vi "Get_Temperature_Percent.vi"(1 "Temperature":dbl, 2 "Setpoint":dbl) -> (0 "Temperature Percent":dbl)   [LabVIEW 2011]
doc: "This VI is a simple macro that determines an absolute percentage value, correlating to the distance from the current setpoint."
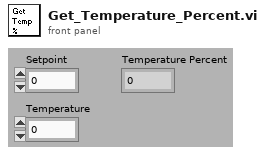
[diagram p1: front panel]
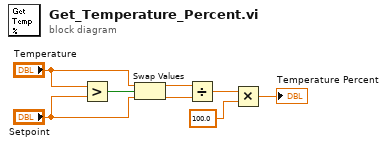
[diagram p0: block diagram]
diagram:
  n1 = Greater?(x="Temperature", y="Setpoint") -> (0:w8:bool)
  n2 = Swap Values(12:"Temperature", 13:w8, 14:"Setpoint") -> (1:w5:dbl, 3:w4:dbl)
  n3 = Divide(x=w5, y=w4) -> (x/y=w3:dbl)
  n4 = Multiply(x=w3, y=100.0) -> (x*y=→"Temperature Percent":dbl)
